vi "Fetch Multi Eval Meas IEM Margin RB Index Results.vi"(8 "error in (no error)":errorcluster, 9 "Result Type (Current)":i32(ring) items=["Current", "Average", "Extreme"], 10 "Instance (1)":T2=1, 11 "VISA resource name":refnum<visa-resource-name>) -> (0 "error out":errorcluster, 1 "Margin RB Index Result":T1, 2 "Reliability":i32, 3 "VISA resource name out":refnum<visa-resource-name>, 4 "Out Of Tolerance":i32)   [LabVIEW 2020, in "Rohde&Schwarz CMWXP NR FR1 Measurement.lvlib"]
doc: "Return resource block indices for current inband emission margins. At these RB indices, the current, average and extreme margins have been detected.\n\nAttributes:\nRSCMWXPNRFR1M_ATTR_FETCH_MULTI_EVAL_MEAS_IEM_MARGIN_RB_INDEX_CURRENT_RESULTS\nRSCMWXPNRFR1M_ATTR_FETCH_MULTI_EVAL_MEAS_IEM_MARGIN_RB_INDEX_AVERAGE_RESULTS\nRSCMWXPNRFR1M_ATTR_FETCH_MULTI_EVAL_MEAS_IEM_MARGIN_RB_INDEX_EXTREME_RESULTS\n\nRemote-control commands:\nFETCh:NRSub:MEAS<i>:MEValuation:IEMission:MARGin:CURRent:RBINdex?\nFETCh:NRSub:MEAS<i>:MEValuation:IEMission:MARGin:AVERage:RBINdex?\nFETCh:NRSub:MEAS<i>:MEValuation:IEMission:MARGin:EXTReme:RBINdex?"
uses:
  <instrlib>/Rohde&Schwarz CMWXP NR FR1 Measurement/Rohde&Schwarz CMWXP NR FR1 Measurement.lvlib
  <instrlib>/Rohde&Schwarz CMWXP NR FR1 Measurement/Private/_Instance.ctl
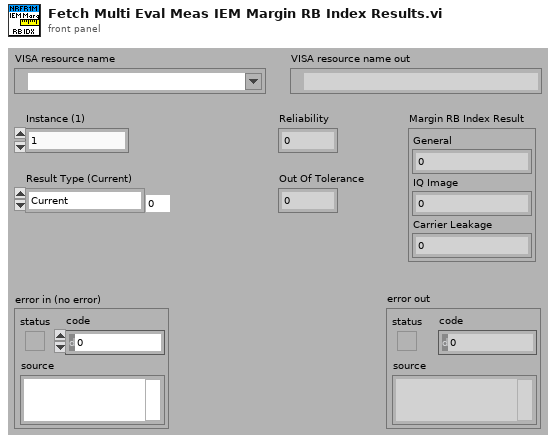
[diagram p1: front panel]
types:
  T1 = cluster{"General":i32, "IQ Image":i32, "Carrier Leakage":i32}
  T2 = typedef "Rohde&Schwarz CMWXP NR FR1 Measurement.lvlib/_Instance.ctl" = i32
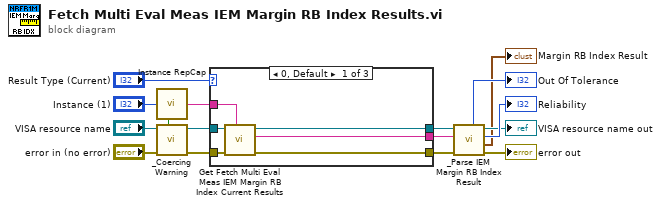
[diagram p0: block diagram]
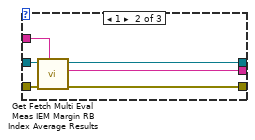
[diagram p2: hidden frame]
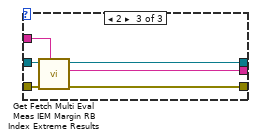
[diagram p3: hidden frame]
diagram:
  n1 = call <instrlib>:"Instance RepCap.vi"("Instance In"="Instance (1)") -> ("In Range?"=w13:bool, "RepCap Identifier Out"=w10:string)  [unwired: 1 in]
  n2 = call <instrlib>:"_Coercing Warning.vi"("In Range?"=w13, "error in (no error)"="error in (no error)", "VISA resource name"="VISA resource name") -> ("error out"=w12:errorcluster, "VISA resource name out"=w11:refnum<visa-resource-name>)  [unwired: 7 in]
  n3 = case shown="0, Default" "Result Type (Current)" {
    tunnel: w12 -> [w22 w28 w34]
    tunnel: w11 -> [w21 w27 w33]
    tunnel: w10 -> [w20 w26 w32]
    tunnel: [w19 w25 w31] -> w8
    tunnel: [w18 w24 w30] -> w7
    tunnel: [w17 w23 w29] -> w6
    frame 0, Default {
      n4 = call "Get Fetch Multi Eval Meas IEM Margin RB Index Current Results"("Repeated Capabilities"=w20, "error in (no error)"=w22, "instrument handle"=w21) -> ("error out"=w17:errorcluster, "Fetch Multi Eval Meas IEM Margin RB Index Current Results"=w18:string, "instrument handle out"=w19:refnum<visa-resource-name>)  [unwired: 6 in]
    }
    frame 1 {
      n5 = call "Get Fetch Multi Eval Meas IEM Margin RB Index Average Results"("Repeated Capabilities"=w26, "error in (no error)"=w28, "instrument handle"=w27) -> ("error out"=w23:errorcluster, "Fetch Multi Eval Meas IEM Margin RB Index Average Results"=w24:string, "instrument handle out"=w25:refnum<visa-resource-name>)  [unwired: 6 in]
    }
    frame 2 {
      n6 = call "Get Fetch Multi Eval Meas IEM Margin RB Index Extreme Results"("Repeated Capabilities"=w32, "error in (no error)"=w34, "instrument handle"=w33) -> ("error out"=w29:errorcluster, "Fetch Multi Eval Meas IEM Margin RB Index Extreme Results"=w30:string, "instrument handle out"=w31:refnum<visa-resource-name>)  [unwired: 6 in]
    }
  }
  n7 = call <instrlib>:"_Parse IEM Margin RB Index Result.vi"("error in (no error)"=w6, "Input String"=w7, "VISA resource name"=w8) -> ("error out"=→"error out":errorcluster, "Margin RB Index Result"=→"Margin RB Index Result":T1, "Reliability"=→"Reliability":i32, "VISA resource name out"=→"VISA resource name out":refnum<visa-resource-name>, "Out Of Tolerance"=→"Out Of Tolerance":i32)  [unwired: 4 in]
